vi "path covt pos array.vi"(1 "path array":T3[](array[typedef]), 2 "recy?":bool) -> (0 "position array":T1[](array[typedef]))   [LabVIEW 2019]
uses:
  ctl/path name.ctl
  ctl/path ctl.ctl
  ctl/position name.ctl
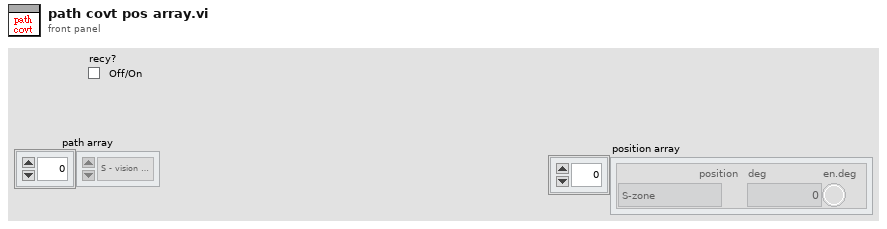
[diagram p1: front panel]
types:
  T1 = typedef "path ctl.ctl" = cluster{"position":T2, "deg":dbl, "en.deg":bool}
  T2 = typedef "position name.ctl" = enum16{"S-zone", "out S", "vision board-vision", "out box", "box catch", "room center", "room right", "room left", "R2", "R4", "only rotate", "out recy", "recycle", "R3", "near board", "box poxition", "R1", "R5", "R1-d", "R5-d", "R3.4", "align center.1", "align center.5", "R2-d", "R2-r", "far center"}
  T3 = typedef "path name.ctl" = enum16{"S - vision board", "vision board - s out", "s out - room center", "room center - R1", "room center - R2", "room center - R3", "room center - R4", "room center - R5", "R1 - room center", "R2 - room center", "R3 - room center", "R4 - room center", "R5 - room center", "room center - S out", "S-out - recycle", "recycle - S-out", "S-out - s", "s - s-out", "board - box", "box - board", "S out - board", "R1 - R1 d", "R5d - R5", "R3.4-R3", "R3 - R3.2", "- align", "- align.5", "R2 - R2.d", "center align"}
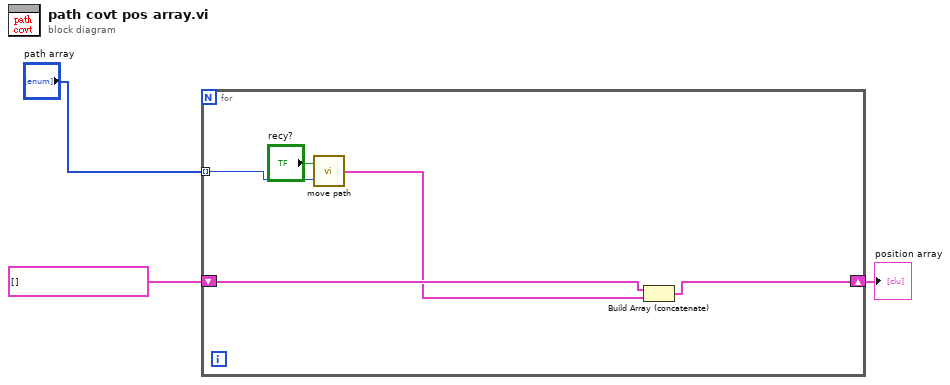
[diagram p0: block diagram]
diagram:
  n1 = for {
    shift-right: [w8] -> w1
    shift-left: T1[] [] ("path array") -> [w7]
    tunnel: "path array" -> [w5] mode=indexing
    n2 = call "move path.vi"("path selsction"=w5, "recy?"="recy?") -> ("path array"=w6:T1[])
    n3 = Build Array (concatenate)(w7, w6) -> (w8:T1[])
  }
  "position array" <- w1
